vi "PH_Sixpack.Reference Search.vi"(0 "i ref in":refnum<vi>, 1 "axis":i32=-1, 4 "Device Error in":errorcluster, 5 "error in":errorcluster) -> (14 "i ref out":refnum<vi>, 18 "Device Error out":errorcluster, 19 "error out":errorcluster)   [LabVIEW 2014, in "PH_Sixpack.lvlib"]
doc: "This VI starts ramping or a reference search."
uses:
  PH_Sixpack.lvlib
  instr.lib/Sixpack/Sixpack - Driver.lvlib
  PH_Basics/PH_Stepmotor_BaseClass/PH_Stepmotor_BaseClass.lvlib
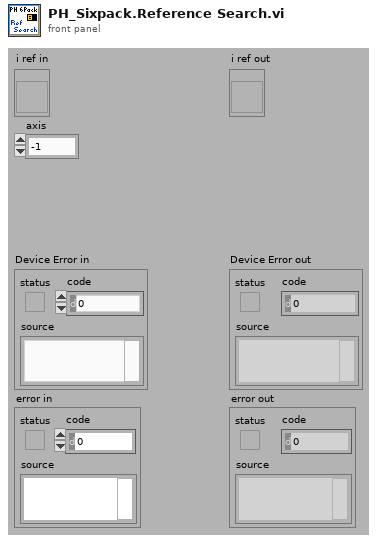
[diagram p1: front panel]
types:
  T1 = typedef "PH_Sixpack.lvlib/PH_Sixpack.i attribute.ctl" = cluster{"Information":cluster{"SixPack ID(0)":u16, "BaudRate(19200)":u16, "COM Port":enum32{"COM1", "COM2", "COM3", "COM4", "COM5", "COM6", "COM7", "COM8", "COM9"}, "HANDLE":i32}, "Serial Number":dbl, "Firmwareversion":dbl, "Axes":T2[], "Status":T14, "Axis to do a RefSearch":i32, "GUI Refs":cluster{"Information":refnum<vi>, "Serial Number":refnum<vi>, "Firmwareversion":refnum<vi>, "Status":refnum<vi>, "Axis to do a RefSearch":refnum<vi>, "Axes Configuration (Sixpack)":refnum<vi>, "Inputs":refnum<vi>, "PeriodicInterval [ms]":refnum<vi>}, "Constructor finished":bool, "Ignore Error":bool}
  T2 = typedef "PH_Sixpack.lvlib/PH_Sixpack.Axis Cluster.ctl" = cluster{"Config":T3, "To set?":cluster{"VmaxAmax":bool, "I max":bool, "VStartVminDivi":bool, "Ref Search Parameter":bool, "Stopswitch Limits":bool, "Axis Parameter":bool, "I Control":bool}}
  T3 = typedef "PH_Sixpack.lvlib/PH_Sixpack.Axis Configuration.ctl" = cluster{"VmaxAmax":T4, "I max (50%)":T5, "VStartVminDivi":T6, "Ref Search Parameter":T7, "Stopswitch Limits":T8, "Axis Parameter":T9, "I Control":T12}
  T4 = typedef "Sixpack - Driver.lvlib/VmaxAmax.ctl" = cluster{"VMax(511)":u16, "AMax(128)":u16}
  T5 = typedef "Sixpack - Driver.lvlib/PeakCurrent.ctl" = dbl
  T6 = typedef "Sixpack - Driver.lvlib/VStartVmin.ctl" = cluster{"VStart(5)":u16, "Vmin(4)":u16, "Div i (2)":enum8{"0", "1", "2", "3"}}
  T7 = typedef "Sixpack - Driver.lvlib/Ref Search Parameter.ctl" = cluster{"VRefMax(100)":u16, "DebouncingTime (22ms)":u8}
  T8 = typedef "Sixpack - Driver.lvlib/Stopswitch Limits.ctl" = cluster{"MinLeft(0)":u16, "MaxRight(1023)":u16}
  T9 = typedef "Sixpack - Driver.lvlib/Motor Parameter.ctl" = cluster{"Poslimit (6400)":u32, "P5 Bits":T10, "P6 Bits":T11}
  T10 = typedef "Sixpack - Driver.lvlib/MotorParameter_P5.ctl" = cluster{"MT_PI":bool, "MT_ROTARY":bool, "MT_AUTONULLCMD":bool, "MT_TESTNULL":bool, "MT_NULLLEFT":bool, "MT_NULLCENTRE":bool, "MT_STOPNULL":bool, "MT_FILTERSWITCH":bool}
  T11 = typedef "Sixpack - Driver.lvlib/MotorParameter_P6.ctl" = cluster{"MT_OPTIMIZEWAY":bool, "MT_FASTREF":bool, "MT_MECHREF":bool, "MT_DELAYTESTNULL":bool, "MT_STOPSOFT":bool, "MT_STOPNOREF":bool, "MT_NULLPOSITIVE":bool, "MUT_STOPFULSTEPS":bool}
  T12 = typedef "Sixpack - Driver.lvlib/Current Control.ctl" = cluster{"PowerDownDelay (500)":u16, "PowerDown (0%)":T13, "Standing (50%)":T13, "Running (75%)":T13, "Accelerating (100%)":T13}
  T13 = typedef "Sixpack - Driver.lvlib/Current.ctl" = enum8{"100%", "75%", "50%", "38%", "25%", "19%", "13%", "9%", "0%"}
  T14 = typedef "PH_Sixpack.lvlib/PH_Sixpack.Status.ctl" = enum32{"None", "Init", "Configure", "configured", "Close", "closed"}
  T15 = typedef "PH_Stepmotor_BaseClass.lvlib/PH_Stepmotor_BaseClass.Axis Attributes.ctl" = cluster{"Settings":T16, "Endswitch?":bool, "DIM Service IDs":T18, "Activity":T19, "Configured?":bool, "Position":cluster{"Current":i32, "Target":i32}, "Position to set":cluster{"New?":bool, "Wanted":i32}, "Stop?":bool, "Reset?":bool, "Move?":bool, "Nothing connected?":bool}
  T16 = typedef "PH_Stepmotor_BaseClass.lvlib/PH_Stepmotor_BaseClass.Axis Settings.ctl" = cluster{"Sign change":bool, "Width":dbl, "Calibration":dbl, "Unit":string, "Motor Type":T17, "Unit Width":string, "Unit CF":string}
  T17 = typedef "PH_Stepmotor_BaseClass.lvlib/PH_Stepmotor_BaseClass.Motor Type.ctl" = enum16{"Unspecific", "OWIS 49.120.2633", "OWIS 49.060.1033", "OWIS 43.040.2558", "Diamond Motion 2200 series", "OWIS 49.120.266B.MV6", "Calorimeter", "Linear Stage 1", "MICOS VT-80", "MICOS VT-80 S", "Standa Rotstage nt0.95A", "PUF RA 320.200", "PUF RA 800.200", "PUF RA 800.400", "PUF RA 400.50", "1324.nn.800.50", "1324.n9c.800.50", "1324.nn.320.200", "1324.nn.400.200", "1324.nn.800.200", "1324.nn.400.50", "1324.8c9c.800.50", "1324.8c9c.400.200"}
  T18 = typedef "PH_Stepmotor_BaseClass.lvlib/PH_Stepmotor_BaseClass.Axis DIM Service IDs.ctl" = cluster{"Settings":i32, "Information":i32}
  T19 = typedef "PH_Stepmotor_BaseClass.lvlib/PH_Stepmotor_BaseClass.Axis Activity.ctl" = enum16{"No Information", "stopped", "running", "Failure", "Alarm", "stopped at backward ES", "stopped at foreward ES"}
  T20 = cluster{"VmaxAmax":bool, "I max":bool, "VStartVminDivi":bool, "Ref Search Parameter":bool, "Stopswitch Limits":bool, "Axis Parameter":bool, "I Control":bool}
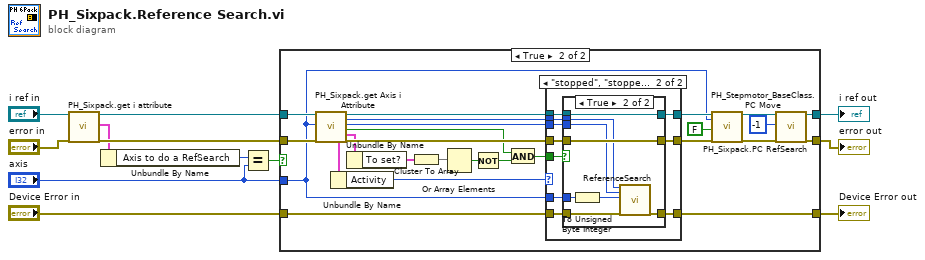
[diagram p0: block diagram]
diagram:
  n1 = call "PH_Sixpack.get i attribute.vi"("i ref in"="i ref in", "error in (no error)"="error in") -> ("i ref out"=w7:refnum<vi>, "i attribute"=w4:T1, "error out"=w5:errorcluster)  [unwired: 15 in]
  n2 = Unbundle By Name(w4) -> ("Axis to do a RefSearch"=w3:i32)
  n3 = Equal?(x=w3, y="axis") -> (x = y?=w1:bool)
  n4 = case shown="True" w1 {
    tunnel: [w13 w41] -> w12
    tunnel: "Device Error in" -> [w13 w40]
    tunnel: [w15 w24] -> w10
    tunnel: [w14 w22] -> w9
    tunnel: w7 -> [w15 w20]
    tunnel: w5 -> [w14 w19]
    tunnel: "axis" -> [_ w18]
    frame False {
    }
    frame True {
      n5 = call "PH_Sixpack.get Axis i Attribute.vi"("VI in"=w20, "Axis"=w18, "error in"=w19) -> ("Axis Base Class Attributes"=w37:T15, "VI out"=w38:refnum<vi>, "HANDLE"=w17:i32, "SixPack ID(0)"=w16:u16, "Axis found?"=w29:bool, "Axis Attributes"=w32:T2, "error out"=w39:errorcluster)  [unwired: 10 in]
      n6 = Unbundle By Name(w37) -> ("Activity"=w36:T19)
      n7 = Unbundle By Name(w32) -> ("To set?"=w35:T20)
      n8 = Cluster To Array(cluster=w35) -> (array=w34:bool[])
      n9 = Or Array Elements(Boolean array=w34) -> (logical OR=w33:bool)
      n10 = Not(x=w33) -> (.not. x?=w31:bool)
      n11 = And(x=w29, y=w31) -> (x .and. y?=w30:bool)
      n12 = case shown="\"stopped\", \"stopped at backward ES\", \"stopped at foreward ES\"" w36 {
        tunnel: [w44 w54] -> w23
        tunnel: [w43 w53] -> w21
        tunnel: [w42 w52] -> w41
        tunnel: w40 -> [w42 w51]
        tunnel: w39 -> [w43 w50]
        tunnel: w38 -> [w44 w49]
        tunnel: w18 -> [_ w48]
        tunnel: w30 -> [_ w47]
        tunnel: w17 -> [_ w46]
        tunnel: w16 -> [_ w45]
        frame "No Information", Default {
        }
        frame "stopped", "stopped at backward ES", "stopped at foreward ES" {
          n13 = case shown="True" w47 {
            tunnel: [w57 w61] -> w54
            tunnel: [w56 w60] -> w53
            tunnel: [w55 w65] -> w52
            tunnel: w51 -> [w55 w64]
            tunnel: w50 -> [w56 w60]
            tunnel: w49 -> [w57 w61]
            tunnel: w48 -> [_ w62]
            tunnel: w46 -> [_ w59]
            tunnel: w45 -> [_ w58]
            frame False {
            }
            frame True {
              n14 = To Unsigned Byte Integer(number=w62) -> (unsigned 8bit integer=w63:u8)
              n15 = call "ReferenceSearch.vi"("handle in"=w59, "UnitAddress(0)"=w58, "MotNr(0)"=w63, "error in"=w64) -> ("error out"=w65:errorcluster)  [unwired: 14 in, 1 out]
            }
          }
        }
      }
      n16 = call "PH_Stepmotor_BaseClass.PC Move.vi"("i ref in"=w23, "axis"=w18, "Move"=FALSE, "error in (no error)"=w21) -> ("i ref out"=w26:refnum<vi>, "error out"=w27:errorcluster)  [unwired: 14 in]
      n17 = call "PH_Sixpack.PC RefSearch.vi"("i ref in"=w26, "axis"=-1, "error in (no error)"=w27) -> ("i ref out"=w24:refnum<vi>, "error out"=w22:errorcluster)  [unwired: 15 in]
    }
  }
  "error out" <- w9
  "i ref out" <- w10
  "Device Error out" <- w12
